vi "Get Child Name[].vi"(8 "error in (no error)":errorcluster, 11 "Doc Class Object[]":refnum<class "Document.lvclass">[](array[class])) -> (0 "error out":errorcluster, 2 "Doc Name[]":string[](array[string]))   [LabVIEW 2016, in "Document.lvclass"]
doc: "Get all Child Window Hwnd."
uses:
  Document.lvclass
  Document.lvclass/Document.ctl
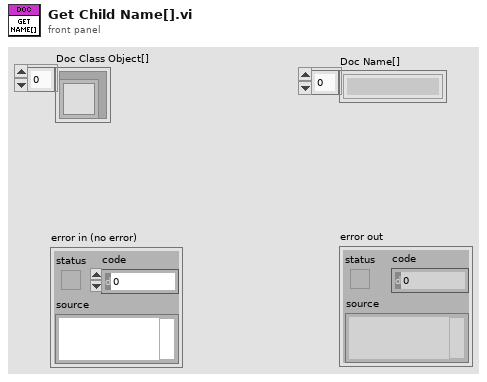
[diagram p1: front panel]
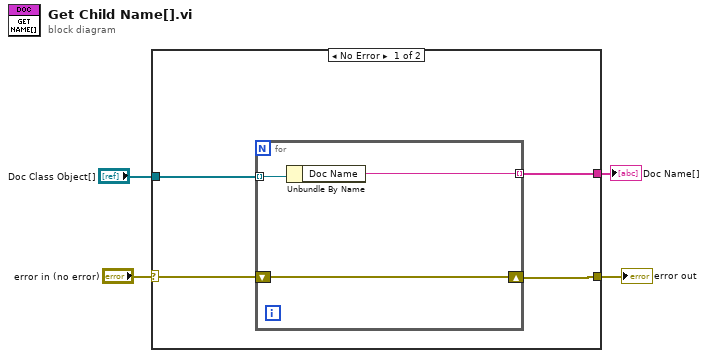
[diagram p0: block diagram]
diagram:
  n1 = case shown="No Error" "error in (no error)" {
    selector: "error in (no error)" -> [w8 w12]
    tunnel: [w7 w12] -> w3
    tunnel: [w6 _] -> w2
    tunnel: "Doc Class Object[]" -> [w5 _]
    frame No Error {
      n2 = for {
        shift-right: [w11] -> w7
        shift-left: w8 -> [w11]
        tunnel: [w9] -> w6 mode=indexing
        tunnel: w5 -> [w10] mode=indexing
        n3 = Unbundle By Name(w10) -> ("Doc Name"=w9:string)
      }
    }
    frame Error {
    }
  }
  "error out" <- w3
  "Doc Name[]" <- w2
